vi "Match Literal Substring.vi"(4 "case matching (sensitive)":T1=enum."system", 6 "offset (0)":i32, 7 "string":string, 8 "literal string":string) -> (0 "offset past match":i32, 1 "found substring":bool, 2 "after substring":string, 3 "match substring":string, 5 "before substring":string)   [LabVIEW 2013, in "TLB` Template.lvlib" / "Tools_String.lvlib"]
uses:
  Tools_String.lvlib
  <vilib>/FTP/util/Case Matching.ctl
  <vilib>/FTP/NI_FTP.lvlib
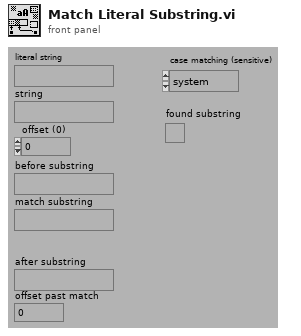
[diagram p1: front panel]
types:
  T1 = typedef "NI_FTP.lvlib/Case Matching.ctl" = enum16{"a != A", "a == A", "system"}
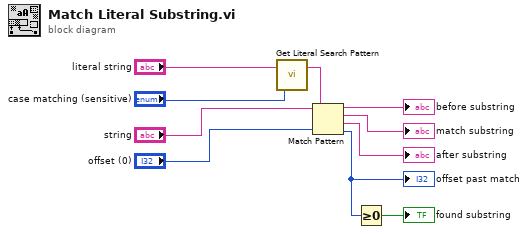
[diagram p0: block diagram]
diagram:
  n1 = call "Get Literal Search Pattern.vi"("case matching (sensitive)"="case matching (sensitive)", "literal string"="literal string") -> ("regular expression"=w4:string)  [unwired: 1 out]
  n2 = Match Pattern(string="string", regular expression=w4, offset (0)="offset (0)") -> (before substring=→"before substring":string, match substring=→"match substring":string, after substring=→"after substring":string, offset past match=w3:i32)
  "offset past match" <- w3
  n3 = Greater Or Equal To 0?(x=w3) -> (x >= 0?=→"found substring":bool)
